vi "Write conversion file.vi"(8 "error in (no error)":errorcluster, 11 "DAQOrcaFlash in":refnum<class "DAQOrcaFlash.lvclass">) -> (0 "error out":errorcluster, 3 "DAQOrcaFlash out":refnum<class "DAQOrcaFlash.lvclass">)   [LabVIEW 2012, in "DAQOrcaFlash.lvclass"]
uses:
  DAQOrcaFlash.lvclass
  DAQOrcaFlash.lvclass/DAQOrcaFlash.ctl
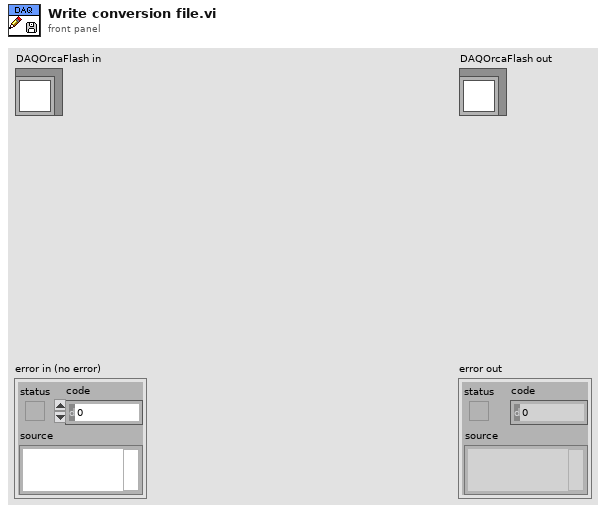
[diagram p1: front panel]
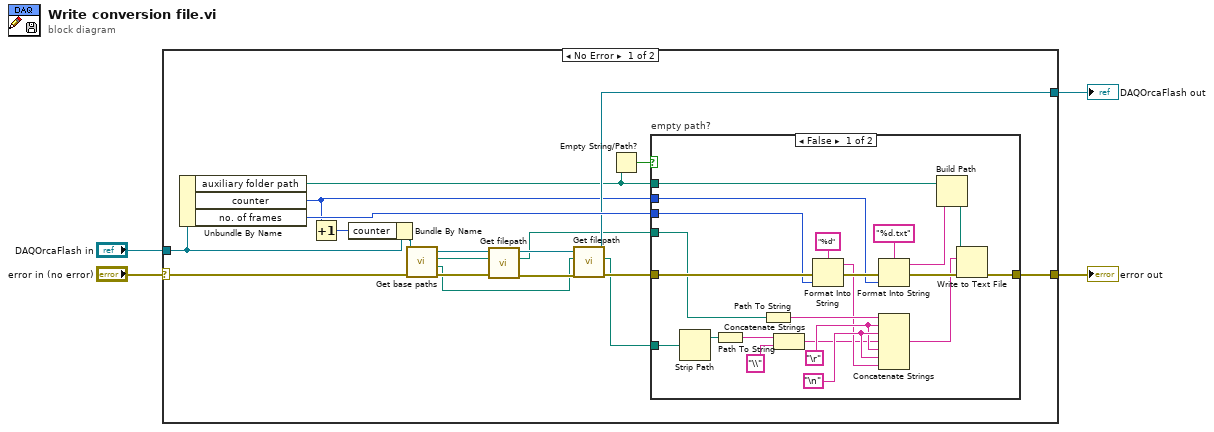
[diagram p0: block diagram]
diagram:
  n1 = case shown="No Error" "error in (no error)" {
    selector: "error in (no error)" -> [w23 w48]
    tunnel: [w20 w48] -> w3
    tunnel: [w18 w47] -> w1
    tunnel: "DAQOrcaFlash in" -> [w19 w47]
    frame No Error {
      n2 = Unbundle By Name(w19) -> ("auxiliary folder path"=w15:path, "counter"=w16:u32, "no. of frames"=w21:i32)
      n3 = Increment(x=w16) -> (x+1=w17:u32)
      n4 = Bundle By Name(cluster=w19, "counter"=w17) -> (w10:refnum<class "DAQOrcaFlash.lvclass">)
      n5 = call-dynamic "Get base paths.vi"("error in (no error)"=w23, "DAQOrcaFlash in"=w10) -> ("error out"=w9:errorcluster, "final conversion folder"=w7:path, "filepath"=w8:path, "DAQOrcaFlash out"=w11:refnum<class "DAQOrcaFlash.lvclass">)  [unwired: 6 in]
      n6 = call "Get filepath.vi"("error in (no error)"=w9, "base path"=w8, "DAQOrcaFlash in"=w11) -> ("error out"=w13:errorcluster, "filepath out"=w6:path, "DAQOrcaFlash out"=w12:refnum<class "DAQOrcaFlash.lvclass">)  [unwired: 6 in]
      n7 = call "Get filepath.vi"("error in (no error)"=w13, "base path"=w7, "DAQOrcaFlash in"=w12) -> ("error out"=w22:errorcluster, "filepath out"=w5:path, "DAQOrcaFlash out"=w18:refnum<class "DAQOrcaFlash.lvclass">)  [unwired: 6 in]
      n8 = Empty String/Path?(string/path=w15) -> (empty?=w14:bool)
      n9 = case "empty path?" shown="False" w14 {
        tunnel: w22 -> [w44 w46]
        tunnel: w21 -> [w42 _]
        tunnel: [w33 w46] -> w20
        tunnel: w6 -> [w32 _]
        tunnel: w16 -> [w31 _]
        tunnel: w15 -> [w28 _]
        tunnel: w5 -> [w27 _]
        frame False {
          w40 = "\n"
          w39 = "\r"
          n10 = Strip Path(path=w27) -> (stripped path=w45:path)  [unwired: 1 out]
          n11 = Path To String(path=w45) -> (string=w25:string)
          n12 = Path To String(path=w32) -> (string=w38:string)
          n13 = Concatenate Strings(w25, "\\" ("string")) -> (w26:string)
          n14 = Format Into String(format string="%d", error in=w44, w42) -> (resulting string=w37:string, error out=w43:errorcluster)  [unwired: 1 in]
          n15 = Format Into String(format string="%d.txt", error in=w43, w31) -> (resulting string=w29:string, error out=w36:errorcluster)  [unwired: 1 in]
          n16 = Concatenate Strings(w38, w39, w40, w26, w39, w40, w37) -> (w34:string)
          n17 = Build Path(base path=w28, name or relative path=w29) -> (appended path=w35:path)
          n18 = Write to Text File(file (use dialog)=w35, text=w34, error in=w36) -> (error out=w33:errorcluster)  [unwired: 1 in, 2 out]
        }
        frame True {
        }
      }
    }
    frame Error {
    }
  }
  "error out" <- w3
  "DAQOrcaFlash out" <- w1
